vi "Close Data Connection.vi"(8 "error in (no error)":errorcluster, 11 "FTP in":refnum<class "FTP.lvclass">) -> (0 "error out":errorcluster, 3 "FTP out":refnum<class "FTP.lvclass">)   [LabVIEW 2017, in "FTP.lvlib" / "FTP.lvclass"]
uses:
  FTP.lvclass
  FTP.lvclass/FTP.ctl
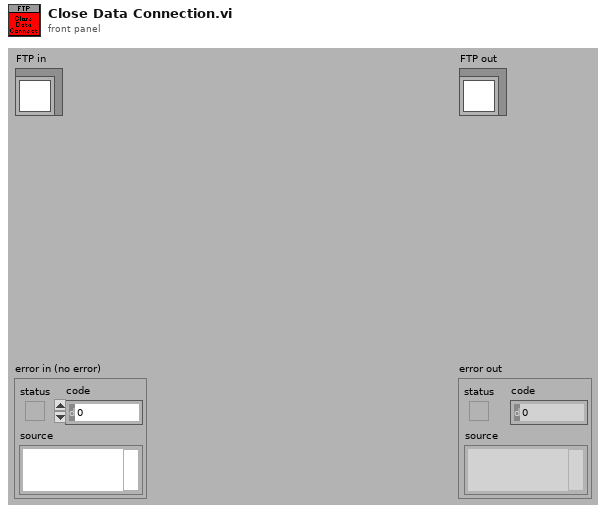
[diagram p1: front panel]
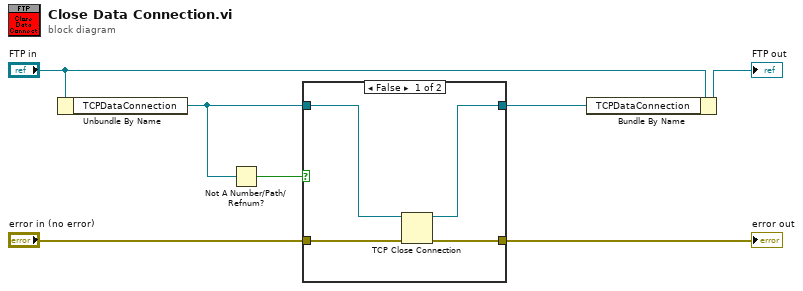
[diagram p0: block diagram]
diagram:
  n1 = Unbundle By Name("FTP in") -> ("TCPDataConnection"=w2:refnum<k5>)
  n2 = Not A Number/Path/Refnum?(number/path/refnum=w2) -> (NaN/Path/Refnum?=w1:bool)
  n3 = case shown="False" w1 {
    tunnel: "error in (no error)" -> [w11 w12]
    tunnel: [w10 w12] -> w6
    tunnel: w2 -> [w9 w13]
    tunnel: [w8 w13] -> w3
    frame False {
      n4 = TCP Close Connection(connection ID=w9, error in (no error)=w11) -> (connection ID out=w8:refnum<k5>, error out=w10:errorcluster)  [unwired: 1 in]
    }
    frame True {
    }
  }
  "error out" <- w6
  n5 = Bundle By Name(cluster="FTP in", "TCPDataConnection"=w3) -> (→"FTP out":refnum<class "FTP.lvclass">)
